vi "EXCEL读取.vi"() -> ()   [LabVIEW 2011]
panel:
  in  "导出sheet位号":i8=1
  in  "存入sheet位号":i8=1
  in  "确定按钮 2":bool
  in  "主页按钮":bool
  out "EXCEL读取":string[][](array[string])
  in  "Excel._Worksheet":refnum<k7>
  in  "路径":path=path "D:/2016_PJT/Auto_Test/PJT_AT/ReceiveData/CompareDataStyle/WW6500K.xlsx"
  in  "Excel._Application":refnum<k7>
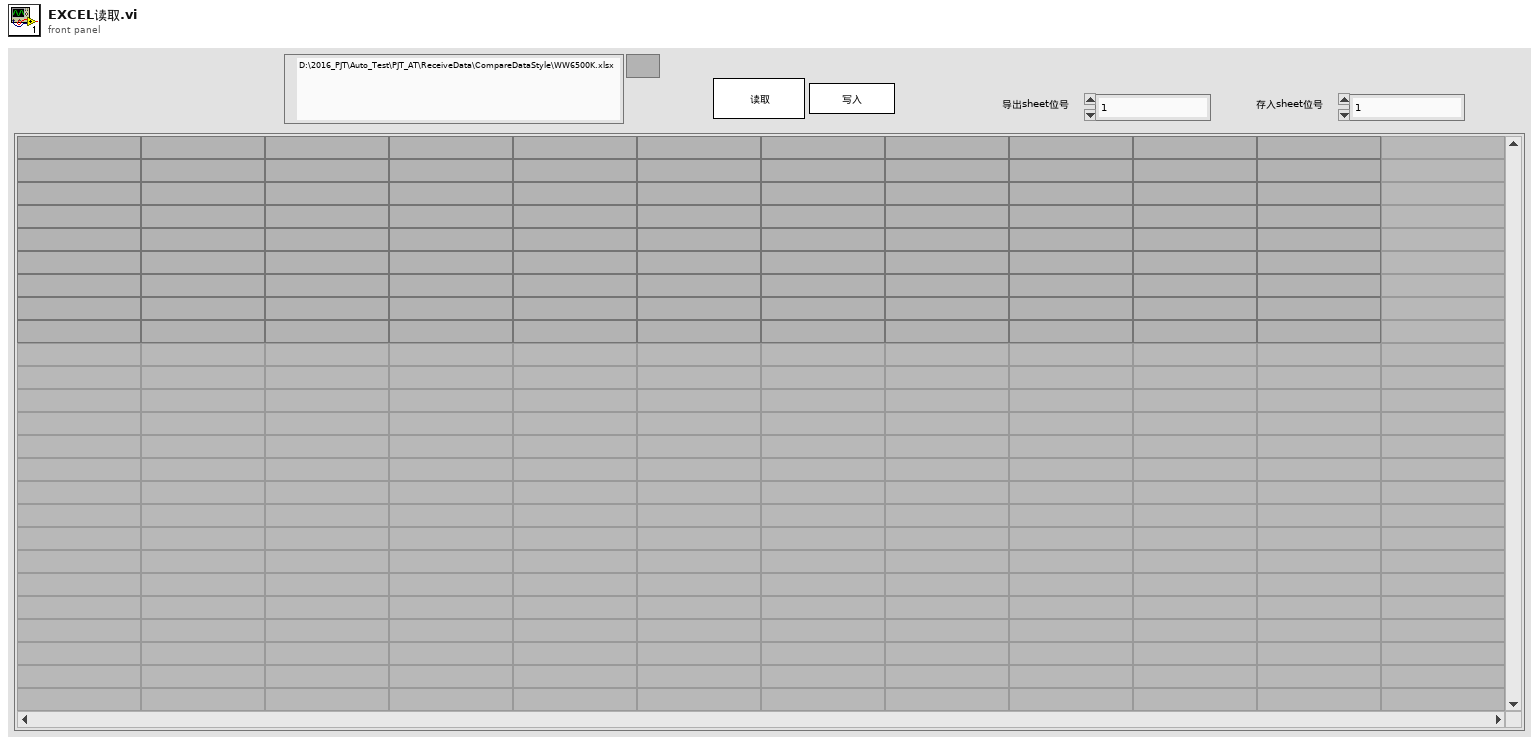
[diagram p1: front panel]
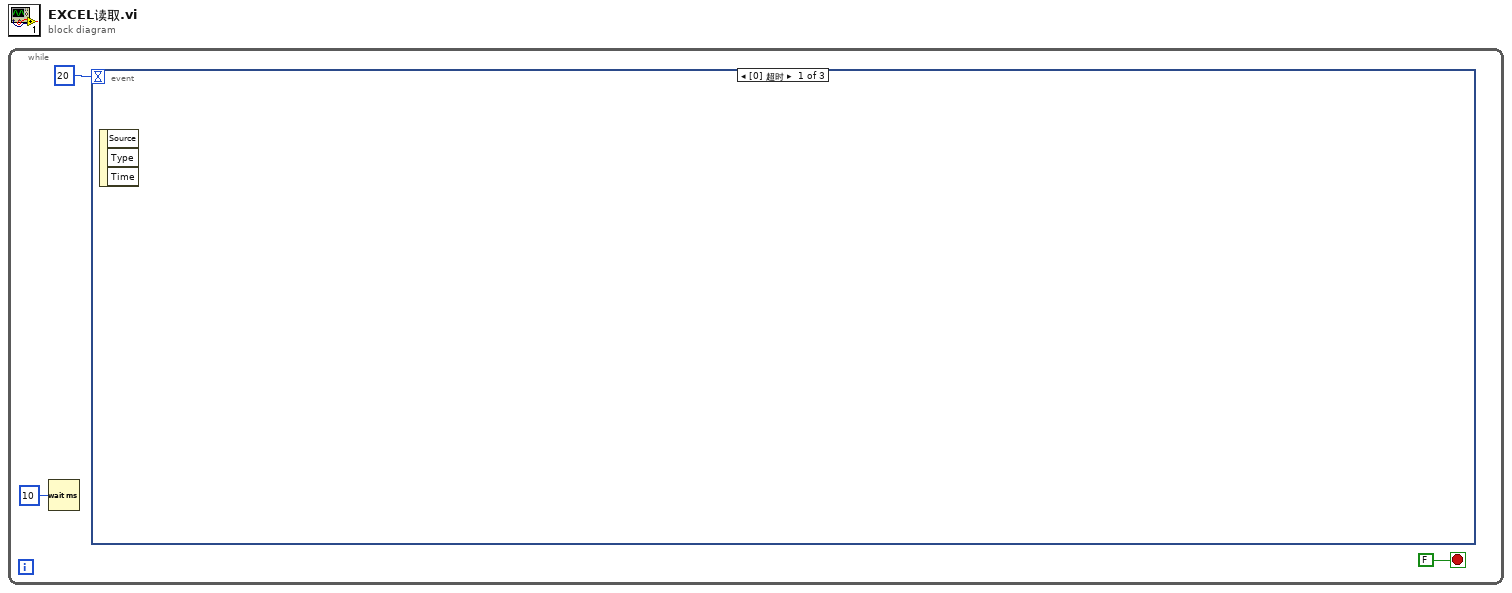
[diagram p0: block diagram]
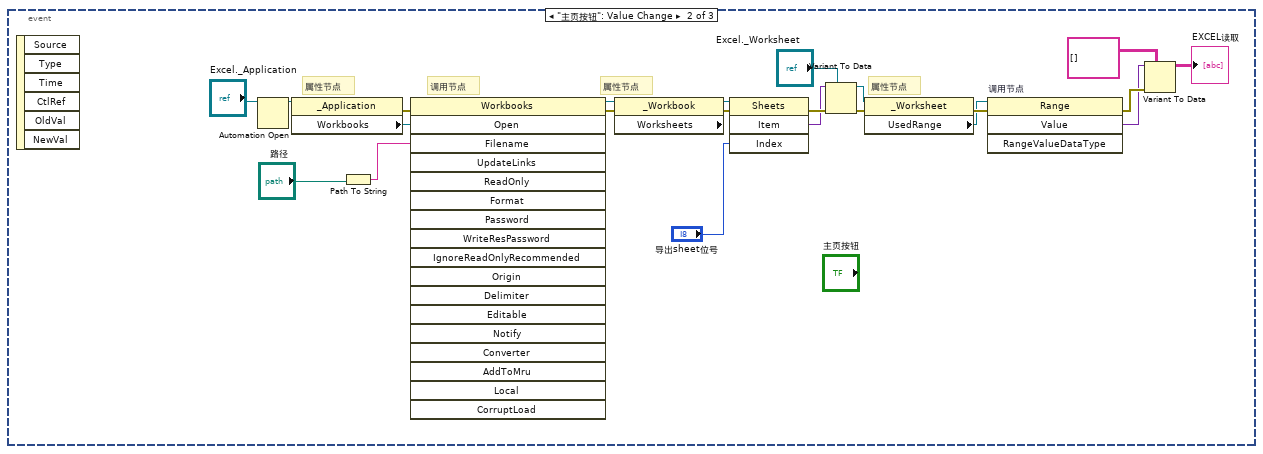
[diagram p2: hidden frame]
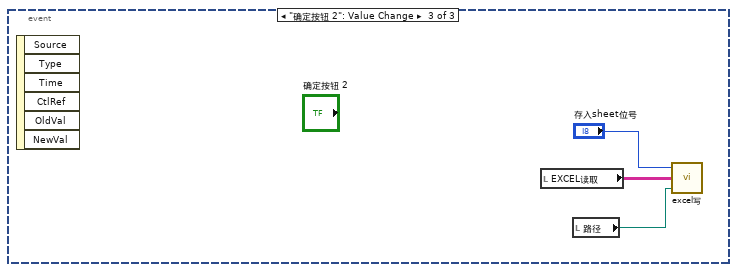
[diagram p3: hidden frame]
diagram:
  n1 = while {
    stop <- FALSE stop-if-true
    n2 = Wait (ms)(milliseconds to wait=u32 10 ("等待时间（毫秒）")) -> ()  [unwired: 1 out]
    n3 = event shown="[0] 超时" {
      selector: _ -> [_ _ _]
      dyn-events: _ -> [_ _ _]
      timeout: 20 -> [_ _ _]
      event Timeout {
        n4 = event-data() -> ()  [unwired: 1 in, 3 out]
      }
      event "主页按钮": Value Change {
        # "属性节点"
        # "属性节点"
        # "属性节点"
        # "调用节点"
        n5 = event-data() -> ()  [unwired: 1 in, 6 out]
        n6 = Automation Open(Automation Refnum="Excel._Application") -> (Automation Refnum=w5:refnum<k7>)  [unwired: 3 in, 1 out]
        n7 = property class="_Application"(reference=w5) -> (error out=w7:errorcluster, "Workbooks"=w6:refnum<k7>)  [unwired: 1 in, 1 out]
        n8 = Path To String(path="路径") -> (string=w9:string)
        n9 = invoke class="Workbooks" method="Open"(reference=w6, error in=w7, "Filename"=w9) -> (error out=w11:errorcluster, "Open"=w10:refnum<k7>)  [unwired: 15 in, 16 out]
        n10 = property class="_Workbook"(reference=w10, error in=w11) -> (error out=w14:errorcluster, "Worksheets"=w13:refnum<k7>)  [unwired: 1 out]
        n11 = invoke class="Sheets" method="Item"(reference=w13, error in=w14, "Index"="导出sheet位号") -> (error out=w16:errorcluster, "Item"=w15:variant)  [unwired: 1 in, 2 out]
        n12 = Variant To Data(error in=w16, type="Excel._Worksheet", Variant=w15) -> (data=w18:refnum<k7>, error out=w19:errorcluster)
        n13 = property class="_Worksheet"(reference=w18, error in=w19) -> (error out=w21:errorcluster, "UsedRange"=w20:refnum<k7>)  [unwired: 1 out]
        n14 = invoke on="调用节点" class="Range" method="Value"(reference=w20, error in=w21) -> (error out=w23:errorcluster, "Value"=w22:variant)  [unwired: 2 in, 2 out]
        n15 = Variant To Data(error in=w23, type=string[][] [], Variant=w22) -> (data=→"EXCEL读取":string[][])  [unwired: 1 out]
      }
      event "确定按钮 2": Value Change {
        n16 = event-data() -> ()  [unwired: 1 in, 6 out]
        n17 = local read "EXCEL读取"() -> (w28:string[][])
        n18 = local read "路径"() -> (w27:path)
        n19 = call "excel写.vi"("路径"=w27, "Table"=w28, "数值"="存入sheet位号") -> ()
      }
    }
  }
